vi "EnviarParametrosArduino.vi"(0 "VISA resource name":refnum<visa-resource-name>, 2 "PARAMETROS DE ENTRADA":T1={"Bandeja Origen"="BANDEJA OK", "Bandeja destino"="BANDEJA NOK", "NUMERO DE ASICS A MOVER"=0, " COORD.ORIGEN X"="00", "COORD.ORIGEN Y"="00", "COORD.DESTINO X"="00", "COORD. DESTINO Y"="00"}, 5 "error in (no error)":errorcluster) -> (14 "VISA resource name 2":refnum<visa-resource-name>, 16 "PARAMETROS DE ENTRADA 2":T1={"Bandeja Origen"="BANDEJA OK", "Bandeja destino"="BANDEJA NOK", "NUMERO DE ASICS A MOVER"=0, " COORD.ORIGEN X"="00", "COORD.ORIGEN Y"="00", "COORD.DESTINO X"="00", "COORD. DESTINO Y"="00"}, 17 "read buffer":string, 18 "enviados":string, 19 "error IO":errorcluster)   [LabVIEW 2019]
uses:
  <vilib>/Utility/error.llb/Error Cluster From Error Code.vi
  <vilib>/ErrorRing/Error Ring.xnode
panel:
  out "return count 2":u32
  out "return count":u32
  out "Parametros enviados = Parametros leídos?":bool
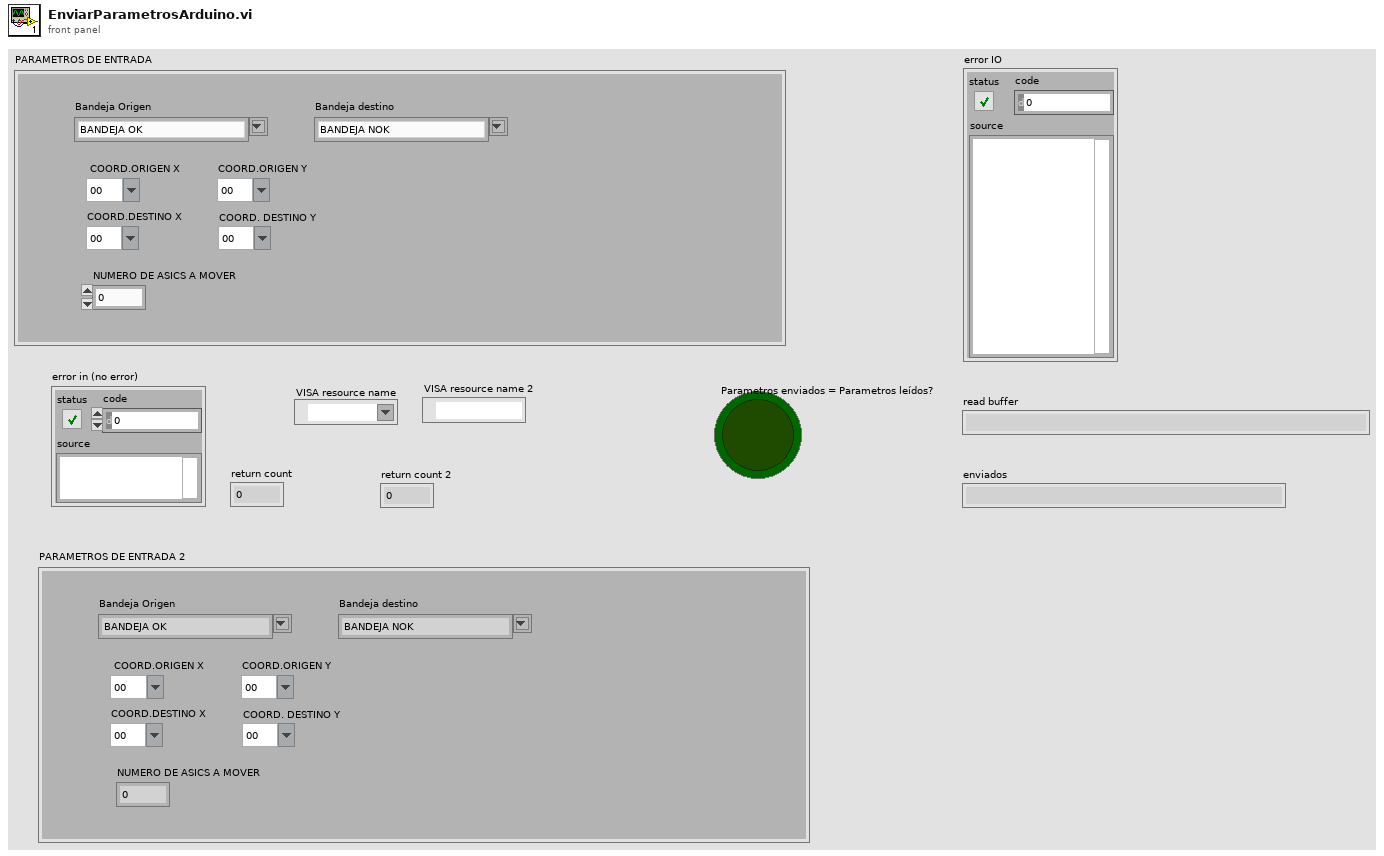
[diagram p1: front panel]
types:
  T1 = typedef "PARÁMETROS.ctl" = cluster{"Bandeja Origen":string, "Bandeja destino":string, "NUMERO DE ASICS A MOVER":i16, " COORD.ORIGEN X":string, "COORD.ORIGEN Y":string, "COORD.DESTINO X":string, "COORD. DESTINO Y":string}
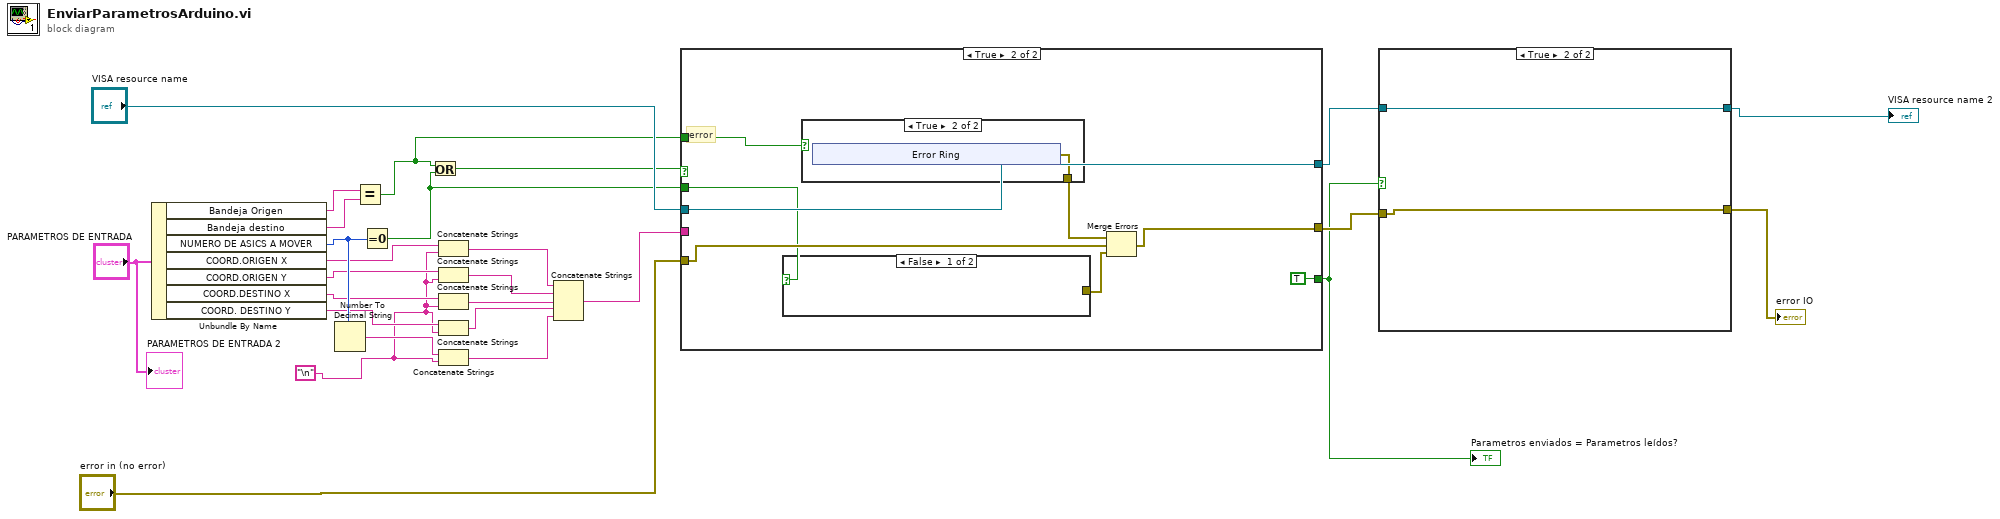
[diagram p0: block diagram]
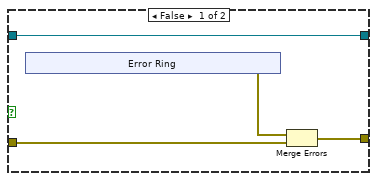
[diagram p2: hidden frame]
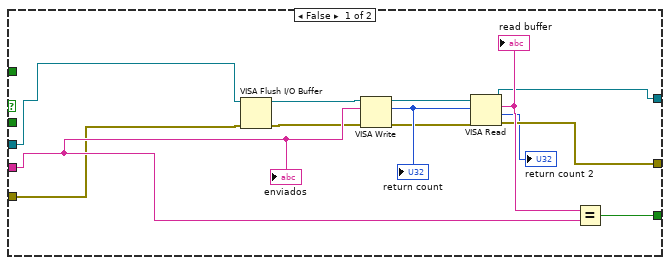
[diagram p3: hidden frame]
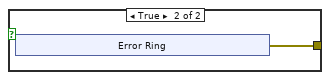
[diagram p4: hidden frame]
diagram:
  w1 = "\n"
  n1 = Unbundle By Name("PARAMETROS DE ENTRADA") -> ("Bandeja Origen"=w20:string, "Bandeja destino"=w19:string, "NUMERO DE ASICS A MOVER"=w18:i16, "COORD.ORIGEN X"=w11:string, "COORD.ORIGEN Y"=w10:string, "COORD.DESTINO X"=w9:string, "COORD. DESTINO Y"=w8:string)
  n2 = Number To Decimal String(number=w18) -> (decimal integer string=w3:string)  [unwired: 1 in]
  n3 = Equal?(x=w20, y=w19) -> (x = y?=w22:bool)
  n4 = Equal To 0?(x=w18) -> (x = 0?=w21:bool)
  n5 = Or(x=w22, y=w21) -> (x .or. y?=w23:bool)
  n6 = Concatenate Strings(w11, w1) -> (w7:string)
  n7 = Concatenate Strings(w10, w1) -> (w6:string)
  n8 = Concatenate Strings(w9, w1) -> (w5:string)
  n9 = Concatenate Strings(w8, w1) -> (w4:string)
  n10 = Concatenate Strings(w3, w1) -> (w2:string)
  n11 = Concatenate Strings(w7, w6, w5, w4, w2) -> (w17:string)
  n12 = case shown="True" w23 {
    tunnel: [w37 w45] -> w16
    tunnel: "error in (no error)" -> [w30 w46]
    tunnel: "VISA resource name" -> [w31 w47]
    tunnel: [w36 w47] -> w14
    tunnel: w22 -> [_ w44]
    tunnel: w21 -> [_ w43]
    tunnel: w17 -> [w38 _]
    tunnel: [w35 TRUE] -> w12
    frame False {
      n13 = VISA Flush I/O Buffer(VISA resource name=w31, error in (no error)=w30) -> (VISA resource name out=w28:refnum<visa-resource-name>, error out=w29:errorcluster)  [unwired: 1 in]
      n14 = VISA Write(VISA resource name=w28, write buffer=w38, error in (no error)=w29) -> (VISA resource name out=w34:refnum<visa-resource-name>, return count=w33:u32, error out=w32:errorcluster)
      "return count" <- w33
      n15 = VISA Read(VISA resource name=w34, byte count=w33, error in (no error)=w32) -> (VISA resource name out=w36:refnum<visa-resource-name>, read buffer=w39:string, return count=→"return count 2":u32, error out=w37:errorcluster)
      "read buffer" <- w39
      n16 = Equal?(x=w39, y=w38) -> (x = y?=w35:bool)
      "enviados" <- w38
    }
    frame True {
      # "error"
      n17 = case shown="False" w43 {
        tunnel: [_ w48] -> w41
        frame False {
        }
        frame True {
          n18 = xnode "Error Ring"() -> ("error out"=w48:errorcluster)
        }
      }
      n19 = case shown="True" w44 {
        tunnel: [_ w54] -> w42
        frame False {
        }
        frame True {
          n20 = xnode "Error Ring"() -> ("error out"=w54:errorcluster)
        }
      }
      n21 = Merge Errors(w42, w46, w41) -> (w45:errorcluster)
    }
  }
  "Parametros enviados = Parametros leídos?" <- w12
  n22 = case shown="True" w12 {
    tunnel: w16 -> [w62 w69]
    tunnel: [w61 w69] -> w15
    tunnel: w14 -> [w60 w70]
    tunnel: [w60 w70] -> w13
    frame False {
      n23 = xnode "Error Ring"() -> ("error out"=w63:errorcluster)
      n24 = Merge Errors(w63, w62) -> (w61:errorcluster)
    }
    frame True {
    }
  }
  "error IO" <- w15
  "VISA resource name 2" <- w13
  "PARAMETROS DE ENTRADA 2" <- "PARAMETROS DE ENTRADA"
